vi "Detect Saccades 2.vi"(8 "error in (no error)":errorcluster, 9 "Config":T1={"Running Stat Time (s)"=10.0, "Thresh Acc Min"=2000.0, "Thresh Acc Mult"=1.3, "Biphasic Condition"=1.5} {"Biphasic Condition" format="%#_13g"; "Thresh Acc Min" format="%#_13g"}, 10 "Sample Rate (Hz)":dbl=500.0, 11 "Velocity Data":dbl[](array[numeric])=[4.667303200298225, 4.909677731146953, 5.2109745814792365, 5.55763581565099, 5.920839247626144, 6.2599375275868905, 6.53696746567776, 6.72865184750785, 6.832732456031344, 6.865145184809078, 6.858206597001612, 6.855560991647909, 6.9019024854844275, 7.042027036538185, 7.301808557734746, 7.67879884433365, 8.162701363544402, 8.739894904566324, 9.381804070066359, 10.060971955287894, 10.76783422583134, 11.502246410072347, 12.262929879380705, 13.045081013541676, 13.853884817610783, 14.695951720056332, 15.571765573591499, 16.488535497561312, 17.454938324359695, 18.484011737786314, 19.593891983853432, 20.806854336741793, 22.151712241900537, 23.654011428085493, 25.337827690951034, 27.230327185694577, 29.362424125147363, 31.75316688648706, 34.39263748770516, 37.23987577100237, 40.20998271205074, 43.18048939513237, 46.018360137909205, 48.61044269433803, 50.91951950237008, 53.06311795006367, 55.36174711261601, 58.34239623139827, 62.72019604358697, 69.31912993124544, 78.92734080431808, 92.11979839547627, 109.07789039502565, 129.463835379339, 152.35306948148417, 176.24888250277527, 199.24480922686814, 219.27781203835607, 234.41475989201246, 243.14123432233515, 244.61162292671878, 238.79626072654116, 226.47186493405752, 209.08996299834854, 188.54095925571488, 166.85076670397655, 145.88590014607087, 127.10744294855878, 111.41329184954873, 99.10408789193212, 89.94838177953986, 83.32435573521803, 78.40945230557072, 74.36256040478978, 70.48301661914127, 66.30206830018594, 61.60225100109197, 56.40307274892831, 50.896616982148316, 45.35594505323262, 40.04915633283459, 35.188143251090374, 30.904438051178893, 27.239307747637383, 24.160247711926996, 21.591099822449937, 19.444244062457226, 17.63526417873216, 16.092631691774315, 14.772784905414664, 13.652421403949939, 12.714696659266576, 11.949486890601628, 11.345398431951562, 10.88883280531385, 10.5770353190049, 10.405836535787293, 10.356779466571126, 10.406311733622601, 10.524935218461192, 10.678830860111066, 10.826005759205444, 10.907035432214682, 10.871451934497463, 10.694375519365607, 10.368230576729, 9.920494644655006, 9.421715176905362, 8.966350342238707, 8.642097141771771, 8.514860672075699, 8.617942426550648, 8.924287001994747, 9.353183534744435, 9.799968965203188, 10.152498912607701, 10.316635671318952, 10.249410666570771, 9.96446844667745, 9.529806688600937, 9.047812081889603, 8.616326801793129, 8.303617903780026, 8.136163116655617, 8.097459448535563, 8.12521569051474, 8.127278177630815, 8.019623108839935, 7.7527652198374994, 7.3178418750367875, 6.743220089832729, 6.091225621655573, 5.4388335182966125, 4.852885740463117, 4.374362223112637, 4.008624562640419, 3.726319072887119, 3.471108403172712, 3.176519977519715, 2.78491418737247, 2.2594461410939903, 1.59493884099372, 0.8181822934693148, -0.026619214287534554, -0.8813264042654012, -1.6754180023234415, -2.342793907914615, -2.8391064532580135, -3.1473600057829927, -3.2704346606176187, -3.2194026522732617, -3.015049071127091, -2.6913407449721714, -2.288963866373292, -1.8552012819132093, -1.4426441696461185, -1.10637493868746, -0.9037185529715961, -0.8855105498645095, -1.0878872191121767, -1.5222387174285608, -2.1642000966113475, -2.948745621863602, -3.774741677175757, -4.521225848850843, -5.0658752955379045, -5.311170309597713, -5.208438257945705, -4.772561349308287, -4.075895907311848, -3.2362701273178054, -2.4080793800097897, -1.7480331896475167, -1.3703588224237055, -1.3200274321352738, -1.5735992621749766, -2.042730927283582, -2.5851998693665657, -3.037924337271747, -3.256090588254791, -3.148166973862299, -2.6984451055504195, -1.9731790520825205, -1.1065567390523348, -0.2681141821144437, 0.37409311669090695, 0.6891756583069366, 0.6155860122500014, 0.17941599326467195, -0.5082906845765738, -1.2803499480545852, -1.9480888478483216, -2.3401497209829145, -2.3440992169137296, -1.9281270895302551, -1.1459474421566647, -0.12830962259723222, 0.9363738210892123, 1.8357991288182767, 2.384599745817786, 2.4666064308939344, 2.054156463248786, 1.220863305309523, 0.12811068784634827, -1.018595010969218, -2.001752664406064, -2.6304649399676983, -2.7869433851410292, -2.4535594735302872, -1.7140485905140306, -0.7334883840388606, 0.27392426391968705, 1.094585023452499, 1.5568403033256075, 1.5611234362432445, 1.0986668385472989, 0.24684742597984943, -0.8452725331409354, -1.9880582489864462, -2.9877533974319324, -3.6879053692364785, -4.00617610589776, -3.9395155261628396, -3.5545628002925387, -2.964302429928681, -2.3045670045288436, -1.7128444883759233, -1.294689818423599, -1.105155718562152, -1.1485119963907628, -1.3895741513688282, -1.7715422803726764, -2.2274763350570232, -2.6932733895783443, -3.113940417779075, -3.45287905028652, -3.70267849231551, -3.8744215557206916, -3.9856590761507915, -4.052808173290114, -4.09332504597233, -4.127471814491399, -4.167454556957223, -4.213014549974331, -4.258926261854726, -4.300292567500452, -4.332119774166569, -4.355168465827725, -4.374979301903575, -4.394294193594332, -4.415209965022706, -4.441144186890184, -4.467481232862541, -4.483248995233593, -4.4855721436010825, -4.4746031408485205, -4.450689654707525, -4.422434151675683, -4.403223628429705, -4.405917482243676, -4.4399518225329295, -4.512143144357493, -4.622080929076186, -4.757550150950738, -4.8958998491602115, -5.008497957121103, -5.0656431974498695, -5.039159628319716, -4.911773985777418, -4.678249782158317]) -> (0 "error out":errorcluster, 3 "Saccades":T2[](array[typedef]))   [LabVIEW 2016]
uses:
  Type Definitions/Saccade Analyser Saccade Data.ctl
  <vilib>/Analysis/NI_AALPro.lvlib
  <vilib>/ptbypt/NI_PtbyPt.lvlib
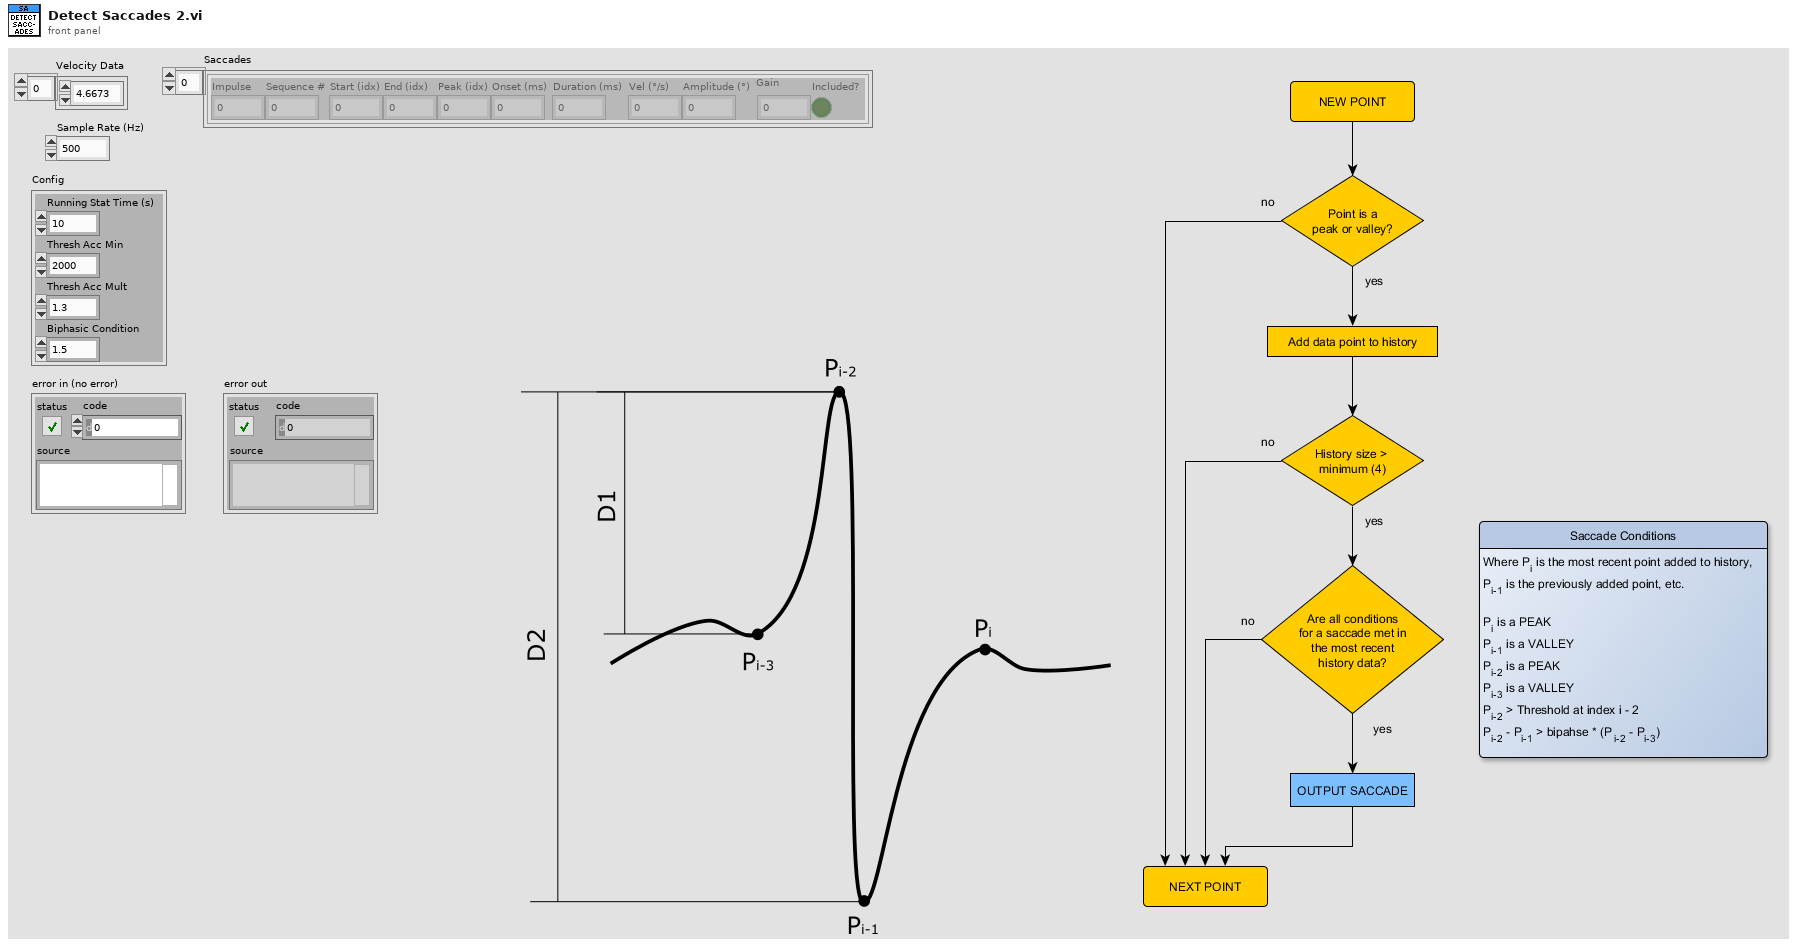
[diagram p1: front panel]
types:
  T1 = cluster{"Running Stat Time (s)":dbl, "Thresh Acc Min":dbl, "Thresh Acc Mult":dbl, "Biphasic Condition":dbl}
  T2 = typedef "Saccade Analyser Saccade Data.ctl" = cluster{"Impulse":i32, "Sequence #":dbl, "Start (idx)":dbl, "End (idx)":dbl, "Peak (idx)":dbl, "Onset (ms)":dbl, "Duration (ms)":dbl, "Vel (°/s)":dbl, "Amplitude (°)":dbl, "Gain":dbl, "Included?":bool}
  T3 = cluster{"Type":enum16{"N/A", "Peak", "Valley"}, "Index":i32, "Value":dbl, "Thresh":dbl}[]
  T4 = cluster{"Type":enum16{"N/A", "Peak", "Valley"}, "Index":i32, "Value":dbl, "Thresh":dbl}
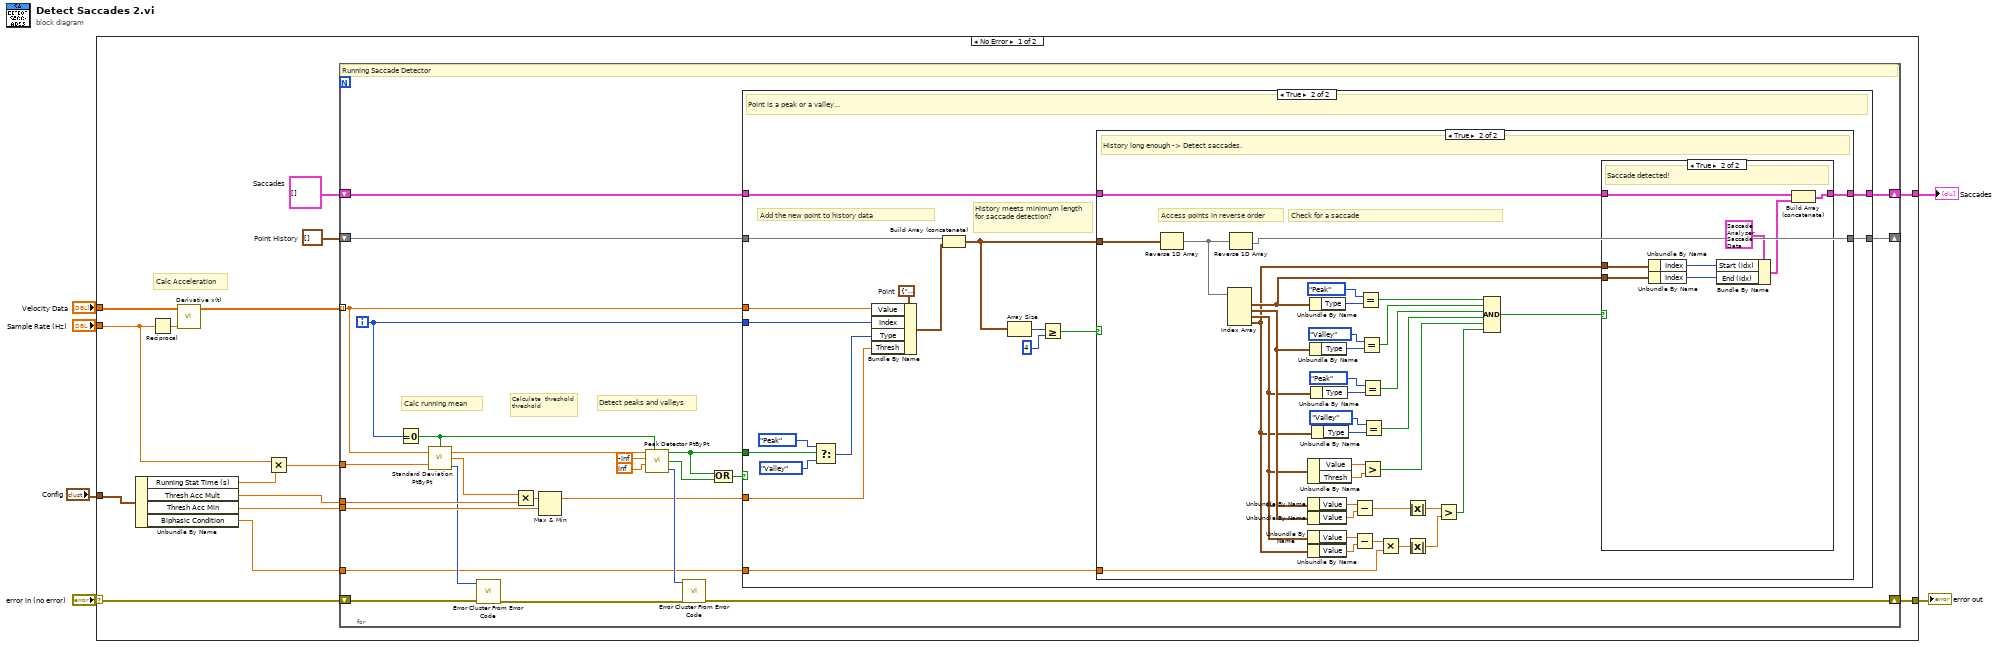
[diagram p0: block diagram]
diagram:
  n1 = case shown="No Error" "error in (no error)" {
    selector: "error in (no error)" -> [w14 w113]
    tunnel: "Velocity Data" -> [w21 _]
    tunnel: "Sample Rate (Hz)" -> [w10 _]
    tunnel: [w17 _] -> w3
    tunnel: [w13 w113] -> w2
    tunnel: "Config" -> [w12 _]
    frame No Error {
      w8 = T3 []  # Point History
      w18 = T2[] []  # Saccades
      # "Calc Acceleration"
      n2 = Unbundle By Name(w12) -> ("Running Stat Time (s)"=w11:dbl, "Thresh Acc Mult"=w15:dbl, "Thresh Acc Min"=w16:dbl, "Biphasic Condition"=w7:dbl)
      n3 = Reciprocal(x=w10) -> (1/x=w20:dbl)
      n4 = call <vilib>:"Derivative x(t).vi"("dt"=w20, "X"=w21) -> ("dX/dt"=w19:dbl[])  [unwired: 8 in, 1 out]
      n5 = Multiply(x=w10, y=w11) -> (x*y=w9:dbl)
      n6 = for {
        tunnel: w19 -> [w29] mode=indexing
        tunnel: w9 -> [w45]
        tunnel: w16 -> [w42]
        shift-right: [w25] -> w17
        shift-left: w18 -> [w26]
        tunnel: w15 -> [w38]
        shift-right: [w35] -> w13
        shift-left: w14 -> [w37]
        shift-right: [w23] -> _
        shift-left: w8 -> [w24]
        tunnel: w7 -> [w22]
        i -> [w28]
        # "Calculate  threshold threshold"
        # "Detect peaks and valleys"
        # "Calc running mean"
        # "Running Saccade Detector"
        n7 = Equal To 0?(x=w28) -> (x = 0?=w44:bool)
        n8 = call <vilib>:"Standard Deviation PtByPt.vi"("x"=w29, "sample length"=w45, "initialize"=w44) -> ("mean"=w41:dbl, "error"=w34:i32)  [unwired: 1 out]
        n9 = call <vilib>:"Error Cluster From Error Code.vi"("error in (no error)"=w37, "error code (0)"=w34) -> ("error out"=w36:errorcluster)  [unwired: 7 in]
        n10 = Multiply(x=w41, y=w38) -> (x*y=w43:dbl)
        n11 = Max & Min(x=w43, y=w42) -> (max(x,y)=w27:dbl)  [unwired: 1 out]
        n12 = call <vilib>:"Peak Detector PtByPt.vi"("x"=w29, "threshold peak"=-inf, "threshold valley"=inf, "initialize"=w44) -> ("peak"=w30:bool, "valley"=w32:bool, "error"=w33:i32)  [unwired: 1 in]
        n13 = call <vilib>:"Error Cluster From Error Code.vi"("error in (no error)"=w36, "error code (0)"=w33) -> ("error out"=w35:errorcluster)  [unwired: 7 in]
        n14 = Compound Arithmetic op=OR(w30, w32) -> (w31:bool)
        n15 = case shown="True" w31 {
          tunnel: w30 -> [_ w65]
          tunnel: w29 -> [_ w61]
          tunnel: w28 -> [_ w60]
          tunnel: w27 -> [_ w58]
          tunnel: w26 -> [w47 w49]
          tunnel: [w47 w48] -> w25
          tunnel: w24 -> [w46 w57]
          tunnel: [w46 w55] -> w23
          tunnel: w22 -> [_ w54]
          frame False {
            # "Point is not a peak or valley. Continue to next point."
          }
          frame True {
            w62 = T4 {"Type"=enum."N/A", "Index"=0, "Value"=0.0, "Thresh"=0.0}  # Point
            # "History meets minimum length for saccade detection?"
            # "Add the new point to history data"
            # "Point is a peak or a valley..."
            n16 = Select(t=enum16{"N/A", "Peak", "Valley"}."Peak" ("Type"), s=w65, f=enum16{"N/A", "Peak", "Valley"}."Valley" ("Type")) -> (s? t:f=w59:enum16{"N/A", "Peak", "Valley"})
            n17 = Bundle By Name(cluster=w62, "Value"=w61, "Index"=w60, "Type"=w59, "Thresh"=w58) -> (w56:T4)
            n18 = Build Array (concatenate)(w57, w56) -> (w53:T3)
            n19 = Array Size(array=w53) -> (size(s)=w52:i32)
            n20 = Greater Or Equal?(x=w52, y=4) -> (x >= y?=w50:bool)
            n21 = case shown="True" w50 {
              tunnel: [w66 w103] -> w55
              tunnel: w54 -> [_ w83]
              tunnel: w53 -> [w66 w73]
              tunnel: w49 -> [w67 w72]
              tunnel: [w67 w71] -> w48
              frame False {
                # "History too short to detect saccades."
              }
              frame True {
                # "Check for a saccade"
                # "Access points in reverse order"
                # "History long enough -> Detect saccades."
                n22 = Reverse 1D Array(array=w73) -> (reversed array=w102:T3)
                n23 = Index Array(array=w102) -> (element #1=w69:T4, element #2=w91:T4, element #3=w86:T4, element #4=w68:T4)  [unwired: 4 in]
                n24 = Reverse 1D Array(array=w102) -> (reversed array=w103:T3)
                n25 = Unbundle By Name(w86) -> ("Value"=w93:dbl, "Thresh"=w92:dbl)
                n26 = Unbundle By Name(w86) -> ("Value"=w90:dbl)
                n27 = Unbundle By Name(w91) -> ("Value"=w89:dbl)
                n28 = Unbundle By Name(w86) -> ("Value"=w87:dbl)
                n29 = Unbundle By Name(w68) -> ("Value"=w88:dbl)
                n30 = Unbundle By Name(w69) -> ("Type"=w100:enum16{"N/A", "Peak", "Valley"})
                n31 = Unbundle By Name(w91) -> ("Type"=w99:enum16{"N/A", "Peak", "Valley"})
                n32 = Unbundle By Name(w86) -> ("Type"=w96:enum16{"N/A", "Peak", "Valley"})
                n33 = Unbundle By Name(w68) -> ("Type"=w95:enum16{"N/A", "Peak", "Valley"})
                n34 = Subtract(x=w90, y=w89) -> (x-y=w85:dbl)
                n35 = Subtract(x=w87, y=w88) -> (x-y=w84:dbl)
                n36 = Equal?(x=enum16{"N/A", "Peak", "Valley"}."Peak" ("Type"), y=w100) -> (x = y?=w79:bool)
                n37 = Equal?(x=enum16{"N/A", "Peak", "Valley"}."Valley" ("Type"), y=w99) -> (x = y?=w78:bool)
                n38 = Equal?(x=enum16{"N/A", "Peak", "Valley"}."Peak" ("Type"), y=w96) -> (x = y?=w77:bool)
                n39 = Greater?(x=w93, y=w92) -> (0:w75:bool)
                n40 = Equal?(x=enum16{"N/A", "Peak", "Valley"}."Valley" ("Type"), y=w95) -> (x = y?=w76:bool)
                n41 = Multiply(x=w84, y=w83) -> (x*y=w82:dbl)
                n42 = Absolute Value(x=w85) -> (abs(x)=w81:dbl)
                n43 = Absolute Value(x=w82) -> (abs(x)=w80:dbl)
                n44 = Greater?(x=w81, y=w80) -> (0:w74:bool)
                n45 = Compound Arithmetic op=AND(w79, w78, w77, w76, w75, w74) -> (w70:bool)
                n46 = case shown="True" w70 {
                  tunnel: w72 -> [w104 w112]
                  tunnel: [w104 w111] -> w71
                  tunnel: w69 -> [_ w107]
                  tunnel: w68 -> [_ w108]
                  frame False {
                    # "No saccade"
                  }
                  frame True {
                    # "Saccade detected!"
                    n47 = Unbundle By Name(w108) -> ("Index"=w105:i32)
                    n48 = Unbundle By Name(w107) -> ("Index"=w106:i32)
                    n49 = Bundle By Name(cluster=T2 {"Impulse"=0, "Sequence #"=0.0, "Start (idx)"=0.0, "End (idx)"=0.0, "Peak (idx)"=0.0, "Onset (ms)"=0.0, "Duration (ms)"=0.0, "Vel (°/s)"=0.0, "Amplitude (°)"=0.0, "Gain"=0.0, "Included?"=FALSE} ("Saccade"), "Start (idx)"=w105, "End (idx)"=w106) -> (w109:T2)
                    n50 = Build Array (concatenate)(w112, w109) -> (w111:T2[])
                  }
                }
              }
            }
          }
        }
      }
    }
    frame Error {
    }
  }
  "error out" <- w2
  "Saccades" <- w3
